vi "CompleteSenslessVi.vi"() -> ()   [LabVIEW 2013]
panel:
  in  "Boolesch":bool
  out "Numerisch":i32
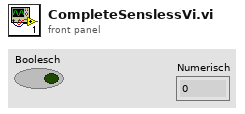
[diagram p1: front panel]
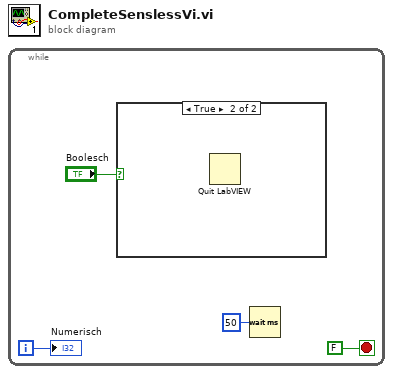
[diagram p0: block diagram]
diagram:
  n1 = while {
    i -> [w4]
    stop <- FALSE stop-if-true
    n2 = case shown="True" "Boolesch" {
      frame False {
      }
      frame True {
        n3 = Quit LabVIEW() -> ()  [unwired: 1 in]
      }
    }
    n4 = Wait (ms)(milliseconds to wait=u32 50 ("Zu wartende ms")) -> ()  [unwired: 1 out]
    "Numerisch" <- w4
  }
